vi "Stop.vi"(8 "error in (no error)":errorcluster, 11 "Sound Card in":refnum<class "Sound Card.lvclass">) -> (0 "error out":errorcluster, 3 "Sound Card out":refnum<class "Sound Card.lvclass">)   [LabVIEW 2010, in "Sound Card.lvclass"]
doc: "Stops any sound playing on the sound card.\n\nThis method is not actually used in the Sound Demo application, but it is included for completeness and future expansion."
uses:
  Sound Card.lvclass
  Sound Card.lvclass/Sound Card.ctl
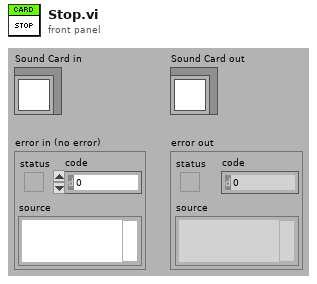
[diagram p1: front panel]
types:
  T1 = typedef "Sound Output Task ID.ctl" = u32
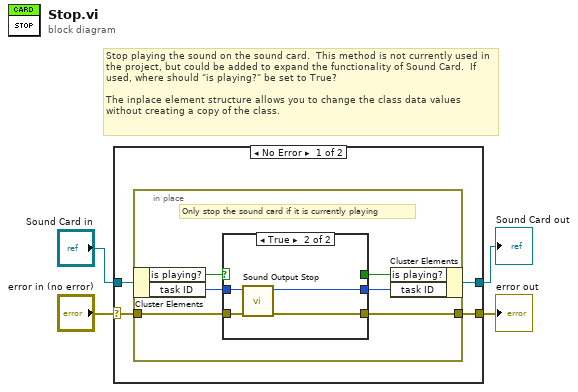
[diagram p0: block diagram]
diagram:
  # "Stop playing the sound on the sound card.  This method is not currently used in the project, but could be added to expand the functionality of Sound Card.  If used, where should \"is playing?\" be set to True?\n\nThe inplace element structure allows you to change the class data values without creating a copy of the class."
  n1 = case shown="No Error" "error in (no error)" {
    selector: "error in (no error)" -> [w8 w23]
    tunnel: [w7 w23] -> w3
    tunnel: "Sound Card in" -> [w6 w22]
    tunnel: [w5 w22] -> w1
    frame No Error {
      n2 = in-place {
        in-place-border: w8 -> [w14]
        in-place-border: [w13] -> w7
        # "Only stop the sound card if it is currently playing"
        n3 = in-place-cluster #1(w6) -> ("is playing?"=w12:bool, "task ID"=w10:T1)
        n4 = case shown="True" w12 {
          selector: w12 -> [w17 _]
          tunnel: w14 -> [w15 w21]
          tunnel: [w15 w20] -> w13
          tunnel: [w17 _] -> w11
          tunnel: w10 -> [w16 w19]
          tunnel: [w16 w18] -> w9
          frame False {
          }
          frame True {
            n5 = call <vilib>:"Sound Output Stop.vi"("error in (no error)"=w21, "task ID"=w19) -> ("error out"=w20:errorcluster, "task ID out"=w18:T1)  [unwired: 8 in]
          }
        }
        n6 = in-place-cluster #1("is playing?"=w11, "task ID"=w9) -> (w5:refnum<class "Sound Card.lvclass">)
      }
    }
    frame Error {
    }
  }
  "error out" <- w3
  "Sound Card out" <- w1
